vi "PageLoad.vi"(8 "error in":errorcluster caption="错误输入（无错误）", 9 "SubPanel*":refnum<vi>, 10 "PanelVIPath":path, 11 "data":string[](array[string])) -> (0 "error out":errorcluster caption="错误输出", 2 "PageNames":string[](array[string]), 3 "VIRefs":refnum<vi>[](array[refnum]))   [LabVIEW 2016, in "PCM PanelSplit.lvclass"]
uses:
  PCM PanelSplit.lvclass
  PanelSplitToolkit/QueueManager.llb/Insert.vi
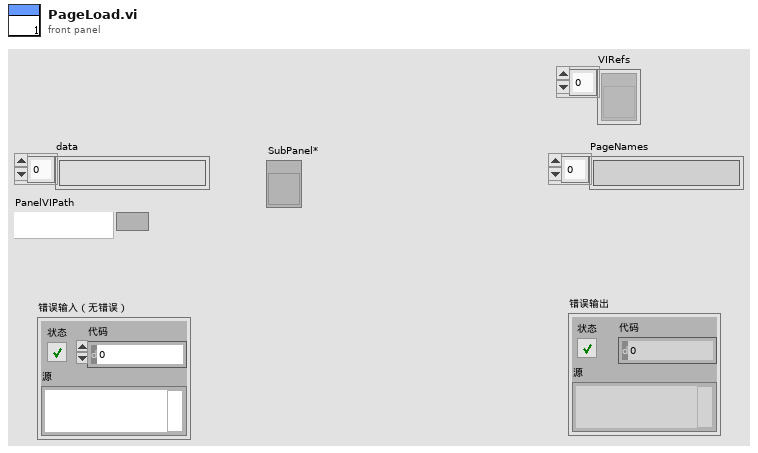
[diagram p1: front panel]
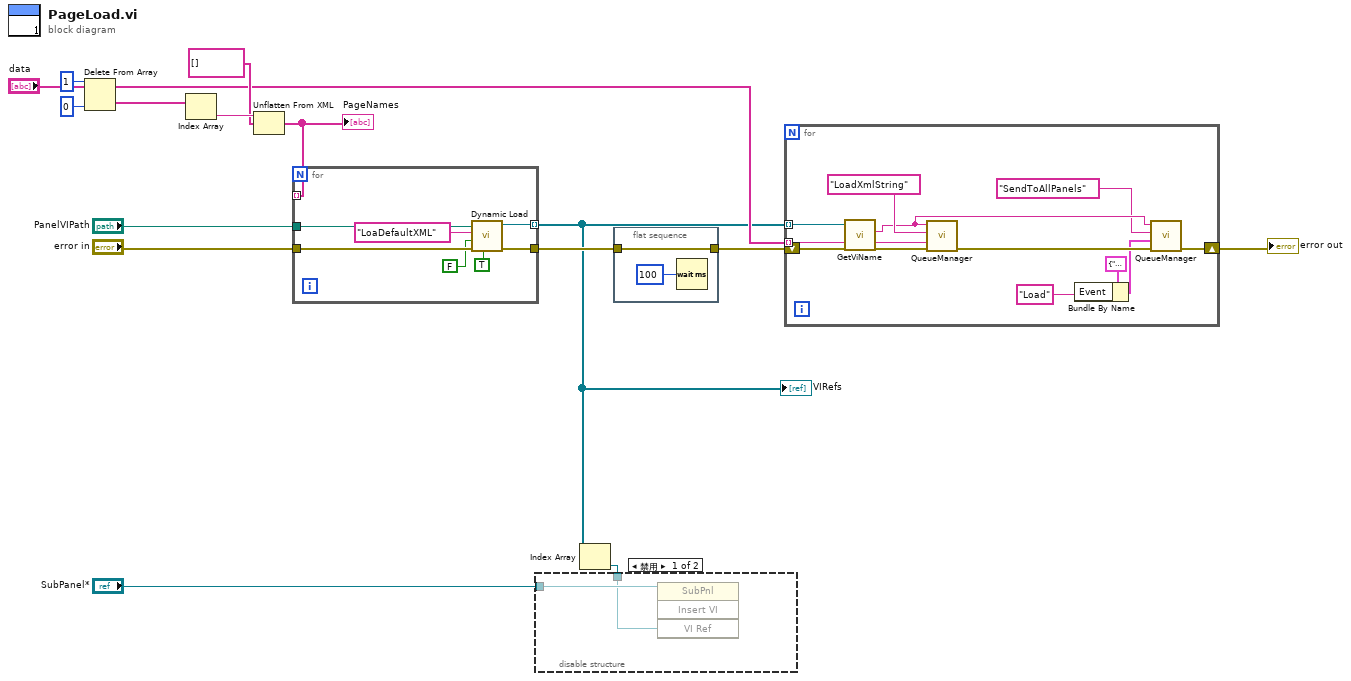
[diagram p0: block diagram]
diagram:
  n1 = Delete From Array(array="data", length=1 ("长度"), index=0 ("索引")) -> (deleted portion=w13:string[], array with subset deleted=w5:string[])
  n2 = Index Array(array=w13) -> (element=w12:string)  [unwired: 1 in]
  n3 = Unflatten From XML(xml string=w12, type=string[] [] ("PageNames")) -> (value=w10:string[])  [unwired: 1 in, 1 out]
  "PageNames" <- w10
  n4 = for {
    tunnel: w10 -> [_] mode=indexing
    tunnel: "PanelVIPath" -> [w23]
    tunnel: [w21] -> w2 mode=indexing
    tunnel: "error in" -> [w20]
    tunnel: [w19] -> w4
    n5 = call "Dynamic Load.vi"("Auto Dispose Ref"=TRUE, "error in"=w20, "CtrlValue"=FALSE ("Auto Dispose Ref"), "CtrlName"="LoaDefaultXML", "Vi Path"=w23) -> ("错误输出"=w19:errorcluster, "vi reference"=w21:refnum<vi>)  [unwired: 5 in]
  }
  "VIRefs" <- w2
  n6 = Index Array(array=w2) -> (element=w6:refnum<vi>)  [unwired: 1 in]
  n7 = disable-structure shown="禁用" {
    disable-tunnel: "SubPanel*" -> [w25 _]
    disable-tunnel: w6 -> [w24 _]
    frame Disabled {
      n8 = invoke class="SubPnl" method="Insert VI"(reference=w25, "VI Ref"=w24) -> ()  [unwired: 2 in, 4 out]
    }
    frame Enabled {
    }
  }
  n9 = flat-sequence {
    tunnel: w4 -> [w27]
    tunnel: [w27] -> w3
    frame #0 {
      n10 = Wait (ms)(milliseconds to wait=u32 100 ("等待时间（毫秒）")) -> ()  [unwired: 1 out]
    }
  }
  n11 = for {
    tunnel: w2 -> [w38] mode=indexing
    tunnel: w5 -> [w37] mode=indexing
    shift-right: [w34] -> w1
    shift-left: w3 -> [w28]
    n12 = call "GetViName.vi"("VI*"=w38) -> ("VI Name"=w33:string)  [unwired: 9 in, 1 out]
    n13 = call-poly "QueueManager.vi"("error in"=w28, "Data"=w37, "Event"="LoadXmlString", "QueueName"=w33) -> ("error out"=w35:errorcluster)  [unwired: 6 in, 1 out]
    n14 = Bundle By Name(cluster=cluster{"Event":string, "Data":variant} {"Event"="", "Data"=variant} ("Send"), "Event"="Load") -> (w30:cluster{"Event":string, "Data":variant})
    n15 = call-poly "QueueManager.vi"("error in"=w35, "Data"=w30, "Event"="SendToAllPanels", "QueueName"=w33) -> ("error out"=w34:errorcluster)  [unwired: 6 in, 1 out]
  }
  "error out" <- w1
